vi "p1.vi"() -> ()   [LabVIEW 2021]
uses:
  <vilib>/Analysis/2dsp.llb/Real FFT.vi
  <vilib>/Analysis/NI_AALPro.lvlib
panel:
  out "Waveform Graph 2":dbl[](graph)
  in  "Nr har 2":dbl(knob) step=1.0 scale=0.0..5.0
  in  "Nr har":dbl(knob) step=1.0 scale=0.0..5.0
  in  "Amp":dbl(knob) scale=0.0..10.0
  out "Waveform Graph":dynamicdata(graph)
  in  "Amp 2":dbl(knob) scale=0.0..10.0
  in  "Amp 1":dbl(knob) scale=0.0..10.0
  in  "Freq":dbl(knob) scale=0.0..5.0 scale format="%#_2g"
  out "Numeric":dbl
  in  "Knob":ext(knob) scale=0.0..1000.0
  in  "stop":bool
  # "signal"
  # "signal char1"
  # "signal char2"
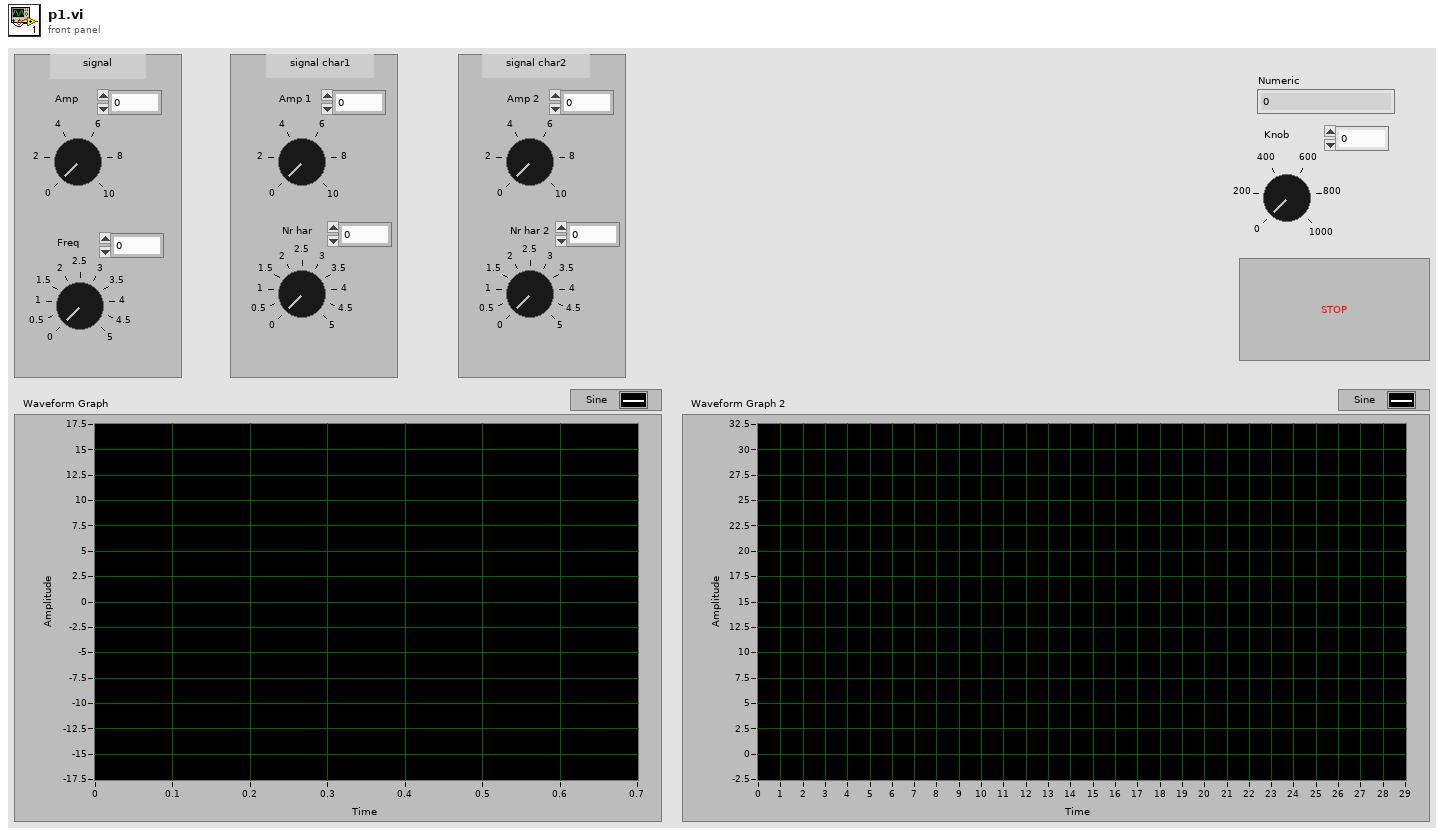
[diagram p1: front panel]
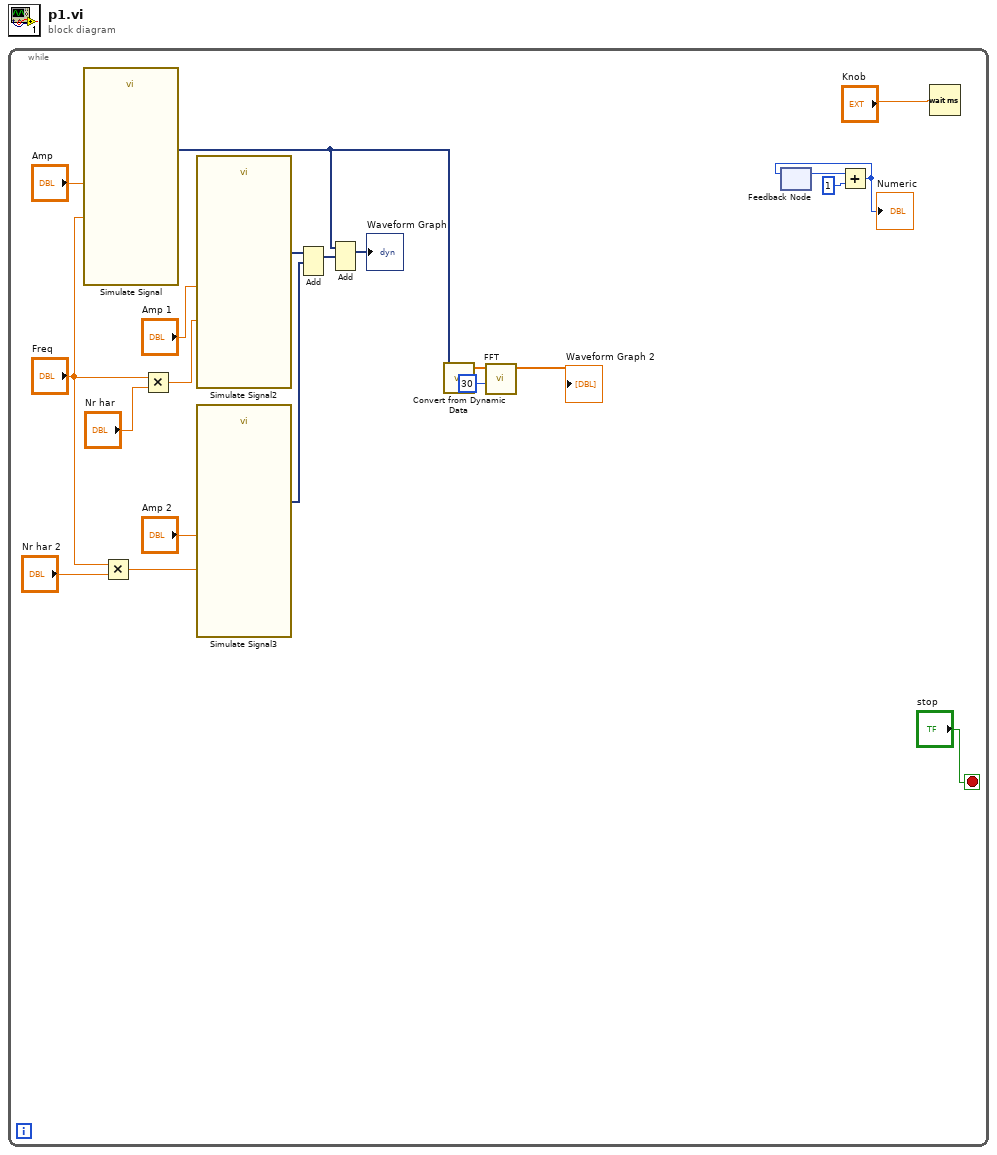
[diagram p0: block diagram]
diagram:
  n1 = while {
    stop <- "stop" stop-if-true
    n2 = call "Simulate Signal"("Frequency"="Freq", "Amplitude"="Amp") -> ("Sine"=w1:dynamicdata)  [unwired: 12 in, 1 out]
    n3 = Multiply(x="Freq", y="Nr har 2") -> (x*y=w9:dbl)
    n4 = Multiply(x="Freq", y="Nr har") -> (x*y=w10:dbl)
    n5 = call "Simulate Signal2"("Frequency"=w10, "Amplitude"="Amp 1") -> ("Sine"=w12:dynamicdata)  [unwired: 12 in, 1 out]
    n6 = call "Simulate Signal3"("Frequency"=w9, "Amplitude"="Amp 2") -> ("Sine"=w13:dynamicdata)  [unwired: 12 in, 1 out]
    n7 = Add(1:w13, 2:w12) -> (0:w11:dynamicdata)  [unwired: 1 in, 1 out]
    n8 = Add(1:w11, 2:w1) -> (0:→"Waveform Graph":dynamicdata)  [unwired: 1 in, 1 out]
    n9 = call "Convert from Dynamic Data"("Dynamic Data Type"=w1) -> ("Array"=w5:dbl[])  [unwired: 3 in]
    n10 = call-poly <vilib>:"FFT.vi"("FFT size"=30, "X"=w5) -> ("FFT {X}"=→"Waveform Graph 2":cdb[])  [unwired: 8 in, 1 out]
    n11 = feedback #1() -> (w17:i32)  [unwired: 1 in]
    n12 = Add(x=w17, y=1) -> (x+y=w18:i32)
    "Numeric" <- w18
    n13 = feedback-in #1(w18) -> ()
    n14 = Wait (ms)(milliseconds to wait="Knob") -> ()  [unwired: 1 out]
  }
